vi "VCS Set Analog Output State.vi"(8 "error in (no error)":errorcluster, 9 "stateValue":u16, 10 "configuration":u16(ring) items=["general Purpose A", "general Purpose B"], 11 "axis in":cluster{"keyHandle":u32, "nodeId":u16}={"keyHandle"=0, "nodeId"=1}) -> (0 "error out":errorcluster, 3 "axis out":cluster{"keyHandle":u32, "nodeId":u16}={"keyHandle"=0, "nodeId"=1})   [LabVIEW 2019, in "maxonEPOS.lvlib"]
doc: "<B>VCS_SetAnalogOutput</B> sets the voltage level of an analog output."
uses:
  Examples/maxonEPOS.lvlib
  Resources/EposCmd64.dll
  Resources/EposCmd.dll
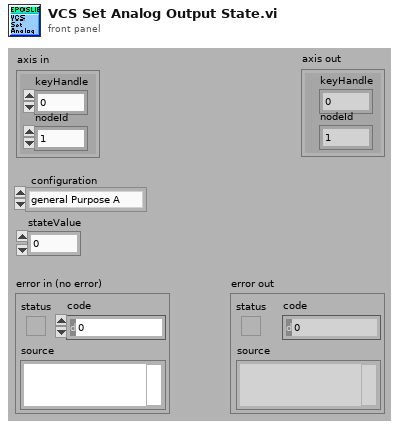
[diagram p1: front panel]
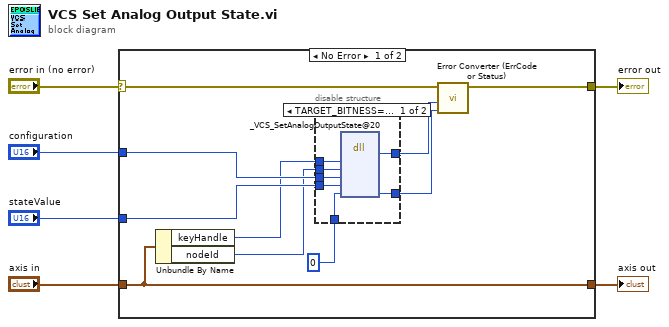
[diagram p0: block diagram]
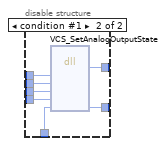
[diagram p2: hidden frame]
diagram:
  n1 = case shown="No Error" "error in (no error)" {
    selector: "error in (no error)" -> [w14 w31]
    tunnel: "axis in" -> [w16 w32]
    tunnel: [w16 w32] -> w5
    tunnel: [w15 w31] -> w4
    tunnel: "stateValue" -> [w12 _]
    tunnel: "configuration" -> [w11 _]
    frame No Error {
      n2 = Unbundle By Name(w16) -> ("keyHandle"=w9:u32, "nodeId"=w10:u16)
      n3 = disable-structure shown="TARGET_BITNESS==32, Standard" {
        disable-tunnel: u32 0 ("pErrorCode") -> [w23 w30]
        disable-tunnel: w12 -> [w22 w29]
        disable-tunnel: w11 -> [w21 w28]
        disable-tunnel: w10 -> [w20 w27]
        disable-tunnel: w9 -> [w19 w26]
        disable-tunnel: [w18 w25] -> w8
        disable-tunnel: [w17 w24] -> w7
        frame condition #0 (active) {
          n4 = dll-call lib="C:/workspace/project/scancon/sw/SSI_Tool/InstrumentsInterfaces/Motordriver/maxon EPOS/Resources/EposCmd.*" fn="_VCS_SetAnalogOutputState@20" ("EposCmd.dll:_VCS_SetAnalogOutput@20")("KeyHandle"=w19, "NodeId"=w20, "Configuration"=w21, "StateValue"=w22, "pErrorCode"=w23) -> ("Rückgabetyp"=w18:i32, "pErrorCode"=w17:u32)  [unwired: 7 in, 2 out]
        }
        frame condition #1 {
          n5 = dll-call lib="C:/Sources/LabView/maxon EPOS/Resources/EposCmd64.*" fn="VCS_SetAnalogOutputState" ("EposCmd.dll:_VCS_SetAnalogOutput@20")("KeyHandle"=w26, "NodeId"=w27, "Configuration"=w28, "StateValue"=w29, "pErrorCode"=w30) -> ("Rückgabetyp"=w25:i32, "pErrorCode"=w24:u32)  [unwired: 7 in, 2 out]
        }
      }
      n6 = call "Error Converter (ErrCode or Status).vi"("error code"=w7, "return type"=w8, "error in (no error)"=w14) -> ("error out"=w15:errorcluster)  [unwired: 7 in]
    }
    frame Error {
    }
  }
  "error out" <- w4
  "axis out" <- w5
